vi "Dashboard Main.vi"() -> ()   [LabVIEW 2017]
uses:
  <vilib>/Utility/miscctls.llb/LVRowAndColumnTypeDef.ctl
  <vilib>/event_ctls.llb/eventvkey.ctl
  <vilib>/Rock Robotics/WPI/Dashboard/WPI_DashboardLogging Global.vi
  <vilib>/Utility/inputDevices.llb/joystickAcquire.vi
  <vilib>/Rock Robotics/Network Tables/NT Read Numeric Array.vi
panel:
  in  "Camera Settings Right":T1={"Frame Rate"=30, "Compression"=30, "Size"=1, "DB Camera Config"=FALSE} {"Frame Rate" scale=1.0..30.0; "Compression" scale=100.0..-1.0; "Size" items=["640x480", "320x240", "160x120"]}
  in  "Camera Name Right":string(combo)="No Camera Selection"
  out "Camera Info":cluster{"Mbps LED":bool, "Mbps":dbl, "fps":dbl} {"fps" format="%#.1g"; "Mbps" format="%#.1g"}
  in  "Camera Settings":T1={"Frame Rate"=30, "Compression"=30, "Size"=1, "DB Camera Config"=FALSE} {"Frame Rate" scale=1.0..30.0; "Compression" scale=100.0..-1.0; "Size" items=["640x480", "320x240", "160x120"]}
  in  "TCP":refnum<k5>
  in  "Rec Mode":enum32{"Stop", "Record", "Playback"}(radio)
  out "Robot IP":string
  out "Image Message":string="Timeout in Camera Communications"
  in  "Dashboard Tab":T2(tab)
  in  "Select Auto":string(combo)="Select Autonomous ..."
  out "NT Connection":bool
  out "MotorChart R":cluster{"Numeric":dbl, "Numeric":dbl}(graph)
  out "MotorChart L":cluster{"Numeric":dbl, "Numeric":dbl}(graph)
  out "MotorSliders R":cluster{"MotorSlide1":dbl, "MotorSlide2":dbl} {"MotorSlide2" scale=-1.0..1.0 scale format="%#_2e"; "MotorSlide1" scale=-1.0..1.0 scale format="%#_2e"}
  out "MotorSliders L":cluster{"MotorSlide1":dbl, "MotorSlide2":dbl} {"MotorSlide2" scale=-1.0..1.0 scale format="%#_2e"; "MotorSlide1" scale=-1.0..1.0 scale format="%#_2e"}
  out "Gyro":dbl(knob) scale=0.0..360.0
  out "JS1 Z":dbl(slide) scale=-1.0..1.0 scale format="%#_2e"
  out "JS1 Graph":cluster{"X":dbl, "Y":dbl}[](graph)
  out "JS1 Buttons":T3
  out "JS2 Z":dbl(slide) scale=-1.0..1.0 scale format="%#_2e"
  out "JS2 Graph":cluster{"X":dbl, "Y":dbl}[](graph)
  out "JS2 Buttons":T3
  out "Mode":T4(ring)=enum."Auto Disabled"
  out "Camera Image Right":T5(plugin-control)
  in  "DB/String 9":string
  in  "DB/String 8":string
  in  "DB/String 7":string
  in  "DB/String 6":string
  in  "DB/String 5":string
  in  "DB/String 4":string
  in  "DB/String 3":string
  in  "DB/String 2":string
  in  "DB/String 1":string
  in  "DB/String 0":string
  in  "DB/Slider 0":dbl(slide) scale=0.0..5.0
  in  "DB/Slider 1":dbl(slide) scale=0.0..5.0
  in  "DB/Slider 2":dbl(slide) scale=0.0..5.0
  in  "DB/Slider 3":dbl(slide) scale=0.0..5.0
  out "DB/LED 3":bool
  out "DB/LED 2":bool
  out "DB/LED 1":bool
  out "DB/LED 0":bool
  in  "DB/Button 3":bool
  in  "DB/Button 2":bool
  in  "DB/Button 1":bool
  in  "DB/Button 0":bool caption="New Name"
  in  "Test Slider":dbl(slide) scale=0.0..100.0 scale format="%#_3g"
  in  "On/Off":bool caption="Solenoid"
  in  "Test Name":u16(ring) items=["Select the test to run..."]
  in  "Test Tree":string(tree)
  in  "Motor":cluster{"Value":dbl, "Enable":bool} {"Value" scale=-1.0..1.0 scale format="%#_3g"}
  out "Progress":T6 {"Test Progress" scale=0.0..100.0}
  in  "Rev/Fwd":cluster{"Forward":bool, "Reverse":bool}
  in  "Test Ring":u16(ring) items=["Monochrome", "Color"]
  out "Cmd Status":string
  in  "Execute Command":bool
  in  "Command Params":string[][](table)
  in  "Command Selection":i32(listbox)
  in  "CheckList":i32(listbox)
  out "Tree":string(tree)
  out "Camera Image":T5(plugin-control)
  out "Background":bool
  in  "Camera Name":string(combo)="No Camera Selection"
  # "HW"
  # "HW"
  # "Joysticks"
  # "Drive Motors"
  # "Front"
  # "Right"
  # "Left"
  # "Back"
  # "This tab is a great place for autonomous settings and robot-specific values.\nPlace controls and indicators inside this tab and match name to\nDashboard Variables on robot. You can also delete this comment."
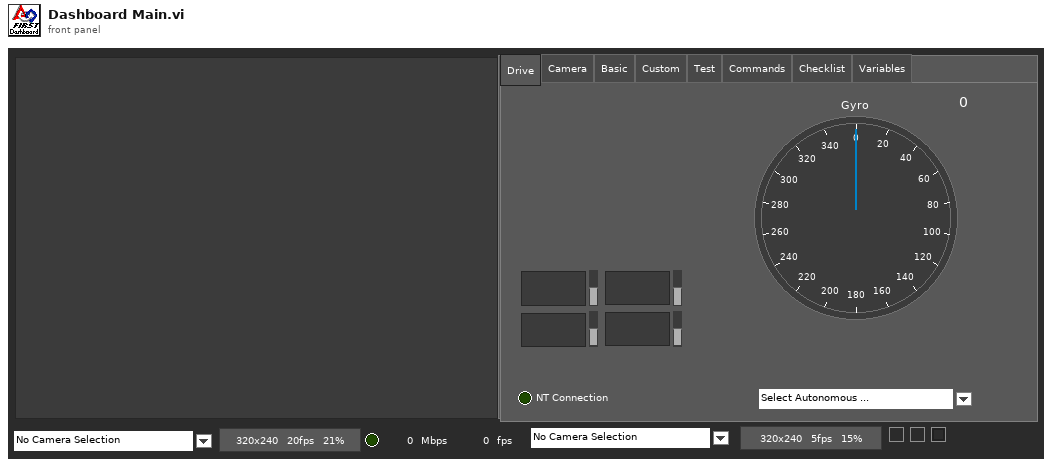
[diagram p1: front panel]
types:
  T1 = cluster{"Frame Rate":i32, "Compression":i32, "Size":u16, "DB Camera Config":bool}
  T2 = enum32{"Drive", "Camera", "Basic", "Custom", "Test", "Commands", "Checklist", "Variables"}
  T3 = cluster{bool, bool, bool, bool, bool, bool, bool, bool, bool, bool, bool, bool}
  T4 = enum8{"Tele-Op Disabled", "Tele-Op Enabled", "Auto Disabled", "Auto Enabled", "Test Disabled", "Test Enabled", "Disconnected", "No Code", "E-Stop"}
  T5 = typedef "IMAQ Image.ctl" = refnum<image>
  T6 = cluster{"Test Progress":u8, "Test Progress Text":string}
  T7 = cluster{"Save Path":path, "Interval (s)":dbl, "Keep":i32}
  T8 = typedef "Image Type" = u32
  T9 = cluster{"IDs":cluster{"RPC field ID":u16, "Unique ID":u16}, "String":string}
  T10 = cluster{"button 1":bool, "button 2":bool, "button 3":bool, "button 4":bool, "button 5":bool, "button 6":bool, "button 7":bool, "button 8":bool, "button 9":bool, "button 10":bool, "button 11":bool, "button 12":bool, "button 13":bool, "button 14":bool, "button 15":bool, "button 16":bool, "button 17":bool, "button 18":bool, "button 19":bool, "button 20":bool, "button 21":bool, "button 22":bool, "button 23":bool, "button 24":bool, "button 25":bool, "button 26":bool, "button 27":bool, "button 28":bool, "button 29":bool, "button 30":bool, "button 31":bool, "button 32":bool}
  T11 = cluster{"Error Strings":string, "Disable Counts":cluster{u16, u16}, "Rail Faults":cluster{u16, u16, u16}, "Robot IP":string, "DB Mode":u8, "Event Info":cluster{"Name":string, "Type":u8, "Number":u16, "Replay":u8}}
  T12 = cluster{"Storage":cluster{"Disk Free":u64, "RAM Block":u32, "RAM free":u32}, "CPU Utilization":cluster{"CPU % ISR":sgl, "CPU % Time Crit":sgl, "CPU % Timed Str":sgl, "CPU % High":sgl, "CPU % Above":sgl, "CPU % Normal":sgl, "CPU % Low":sgl}, "CAN":cluster{"% Bus Utilization":sgl, "Bus Off Cnt":u32, "TX_FIFO Full Cnt":u32, "Receive Error Cnt":u8, "Transmit Error Cnt":u8}, "HID":cluster{"HID Outputs":u32, "Rumble Low":u16, "Rumble High":u16}[]}
  T13 = cluster{"Status bits":cluster{"Test Mode":bool, "Autonomous":bool, "Enabled":bool, "Code Start":bool, "Brownout":bool, "Reserved 2":bool, "Reserved 3":bool, "E-Stop":bool}, "Code Trace":cluster{"Disabled":bool, "TeleOp":bool, "Auto":bool, "Test":bool}, "Controller Type":enum16{"unknown", "cRIO", "roboRio"}, "Code?":enum16{"unknown", "noCode", "code"}, "Battery V":dbl}
  T14 = cluster{"Control Bits":cluster{"TestMode":bool, "Autonomous":bool, "Enabled":bool, "FMS Present":bool, bool, bool, bool, "E-Stop":bool}, "Team Station ":u8, "Countdown":sgl, "Joystick Values":cluster{"Axes":dbl[], "Buttons":bool[], "POVs":i16[]}[]}
  T15 = cluster{"Axes":dbl[], "Buttons":bool[], "POVs":i16[]}[]
  T16 = cluster{"Axes":dbl[], "Buttons":bool[], "POVs":i16[]}
  T17 = cluster{"Buttons[0]":bool, "Buttons[1]":bool, "Buttons[2]":bool, "Buttons[3]":bool, "Buttons[4]":bool, "Buttons[5]":bool, "Buttons[6]":bool, "Buttons[7]":bool, "Buttons[8]":bool, "Buttons[9]":bool, "Buttons[10]":bool, "Buttons[11]":bool}
  T18 = cluster{"Camera Image":refnum<vi>, "Dashboard Tab":refnum<vi>, "Background":refnum<vi>, "Rec Mode":refnum<vi>, "Test Slider":refnum<vi>, "On/Off ":refnum<vi>, "Test Ring":refnum<vi>, "Rev/Fwd":refnum<vi>, "Test Name":refnum<vi>, "Motor":refnum<vi>, "Progress":refnum<vi>, "CheckList":refnum<vi>, "Tree":refnum<vi>, "Test Tree":refnum<vi>, "Command Params":refnum<vi>, "Command Selection":refnum<vi>, "Execute Command":refnum<vi>, "Cmd Status":refnum<vi>, "Camera Settings":refnum<vi>, "Camera Name":refnum<vi>, "Camera Info":refnum<vi>, "Camera Settings Right":refnum<vi>, "Camera Name Right":refnum<vi>, "Camera Image Right":refnum<vi>}
  T19 = cluster{"Camera Name Right":string, string, "Saved DB Images Info":cluster{"Save Path":path, "Interval (s)":dbl, "Keep":i32}}
  T20 = cluster{"Camera Name":string, string, "Saved DB Images Info":cluster{"Save Path":path, "Interval (s)":dbl, "Keep":i32}}
  T21 = cluster{"Operation":enum16{"Update", "Clear"}, "Color Box":u32}[]
  T22 = typedef "eventvkey.ctl" = enum16{"ASCII", "Enter", "Return", "Shift", "Ctrl", "Alt", "Cmd", "Opt", "Caps", "NumLock", "Clear", "Break", "Up", "Down", "Left", "Right", "Insert", "Delete", "Home", "End", "PageUp", "PageDown", "Escape", "Help", "Pause", "ScrollLock", "F1", "F2", "F3", "F4", "F5", "F6", "F7", "F8", "F9", "F10", "F11", "F12", "F13", "F14", "F15", "F16", "F17", "F18", "F19", "F20", "F21", "F22", "F23", "F24", "Play", "VolumeUp", "VolumeDown", "Mute", "Two Byte Char"}
  T23 = cluster{"Image Size":bool, "Image Type":bool, "Pixel Value":bool, "ROI Information":bool, "Zoom Factor":bool}
  T24 = cluster{"Operation":enum16{"Update", "Clear"}, "Color Box":u32}
  T25 = typedef "LVRowAndColumnTypeDef.ctl" = cluster{"Row":i32, "Column":i32}
  T26 = cluster{"Shift":bool, "Ctrl":bool, "Alt":bool, "Cmd":bool, "Opt":bool}
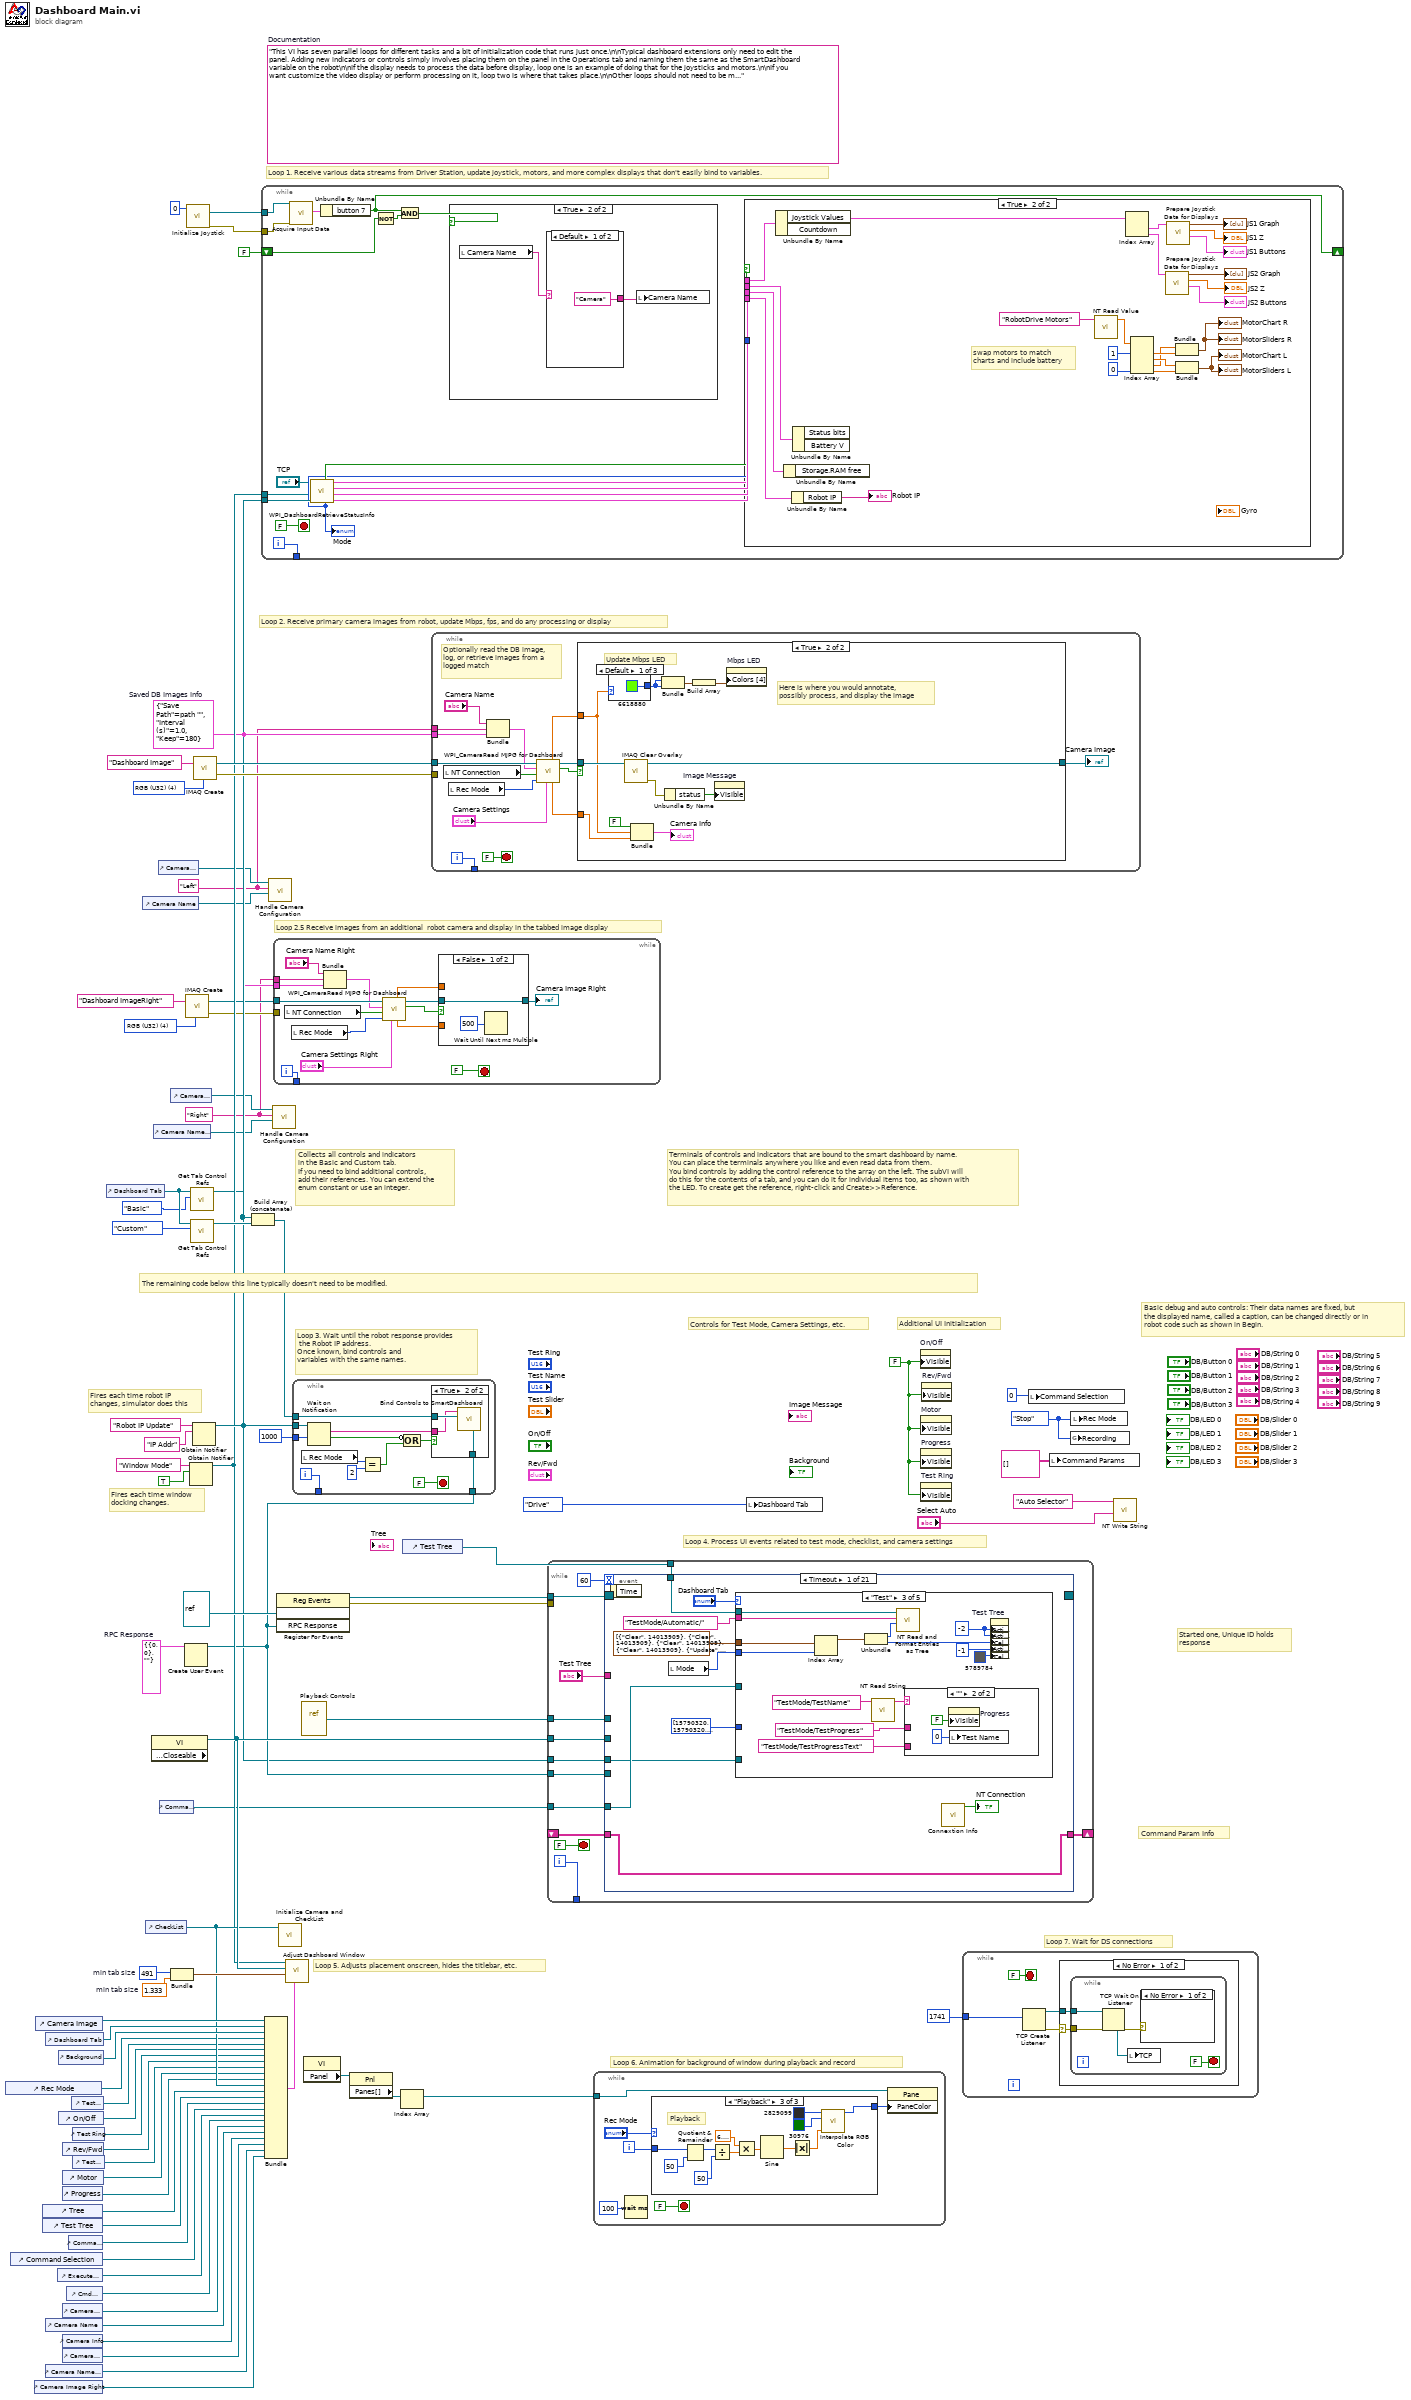
[diagram p0: block diagram]
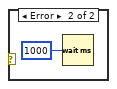
[diagram p3: hidden frame]
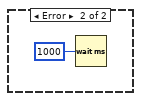
[diagram p4: hidden frame]
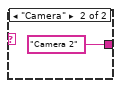
[diagram p6: hidden frame]
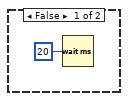
[diagram p7: hidden frame]
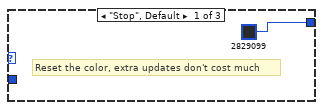
[diagram p8: hidden frame]
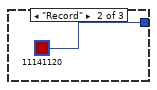
[diagram p9: hidden frame]
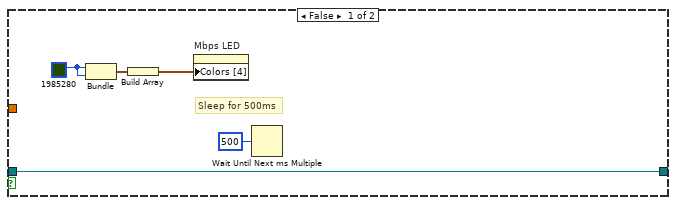
[diagram p11: hidden frame]
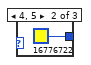
[diagram p12: hidden frame]
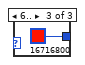
[diagram p13: hidden frame]
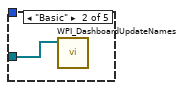
[diagram p15: hidden frame]
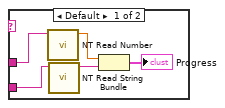
[diagram p16: hidden frame]
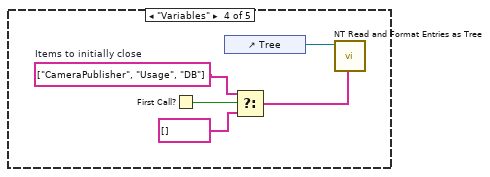
[diagram p17: hidden frame]
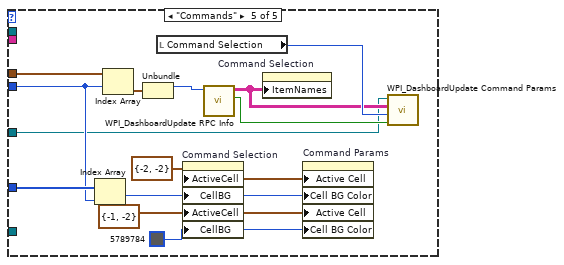
[diagram p18: hidden frame]
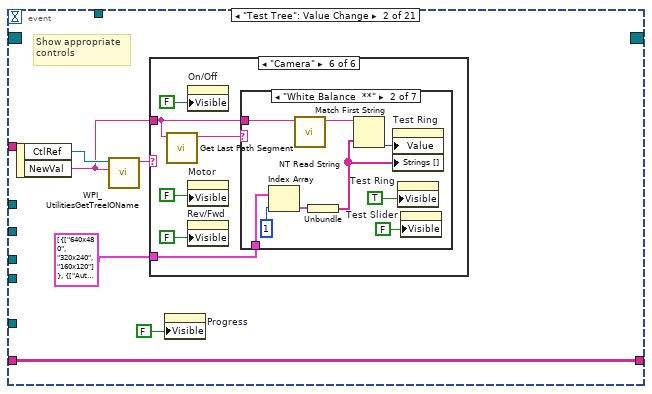
[diagram p19: hidden frame]
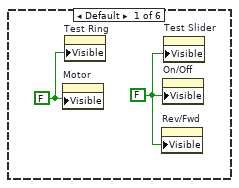
[diagram p20: hidden frame]
diagram:
  w7 = T7 {"Save Path"=path "", "Interval (s)"=1.0, "Keep"=180}  # Saved DB Images Info
  w6 = "Right"
  w5 = "Left"
  w17 = T8 4 items=["Grayscale (U8)", "Grayscale (I16)", "Grayscale (SGL)", "Complex (CSG)", "RGB (U32)", "HSL (U32)", "RGB (U64)"] ("Image Type")
  w33 = T9 {"IDs"={"RPC field ID"=0, "Unique ID"=0}, "String"=""}  # RPC Response
  w56 = 491  # min tab size
  w55 = 1.333  # min tab size
  w63 = enum32{"Stop", "Record", "Playback"}."Stop" ("Rec Mode")
  w40 = FALSE ("Visible")
  (unwired) "This VI has seven parallel loops for different tasks and a bit of initialization code that runs just once.\n\nTypical dashboard extensions only need to edit the panel. Adding new indicators or controls simply involves placing them on the panel in the Operations tab and naming them the same as the SmartDashboard variable on the robot\n\nIf the display needs to process the data before display, loop one is an example of doing that for the joysticks and motors.\n\nIf you want customize the video display or perform processing on it, loop two is where that takes place.\n\nOther loops should not need to be modified. They are pretty standard, and document the task they perform."  # Documentation
  w80 = T8 4 items=["Grayscale (U8)", "Grayscale (I16)", "Grayscale (SGL)", "Complex (CSG)", "RGB (U32)", "HSL (U32)", "RGB (U64)"] ("Image Type")
  # "Loop 2.5 Receive images from an additional  robot camera and display in the tabbed image display"
  # "Command Param Info"
  # "Started one, Unique ID holds\nresponse"
  # "Loop 7. Wait for DS connections"
  # "Basic debug and auto controls: Their data names are fixed, but\nthe displayed name, called a caption, can be changed directly or in\nrobot code such as shown in Begin."
  # "Controls for Test Mode, Camera Settings, etc."
  # "Additional UI Initialization"
  # "Loop 6. Animation for background of window during playback and record"
  # "Fires each time robot IP\nchanges, simulator does this"
  # "Fires each time window\ndocking changes."
  # "Collects all controls and indicators\nin the Basic and Custom tab.\nIf you need to bind additional controls,\nadd their references. You can extend the\nenum constant or use an integer."
  # "The remaining code below this line typically doesn't need to be modified."
  # "Loop 4. Process UI events related to test mode, checklist, and camera settings"
  # "Terminals of controls and indicators that are bound to the smart dashboard by name.\nYou can place the terminals anywhere you like and even read data from them.\nYou bind controls by adding the control reference to the array on the left. The subVI will\ndo this for the contents of a tab, and you can do it for individual items too, as shown with\nthe LED. To create get the reference, right-click and Create>>Reference."
  # "Loop 3. Wait until the robot response provides\n the Robot IP address.\nOnce known, bind controls and\nvariables with the same names."
  # "Loop 5. Adjusts placement onscreen, hides the titlebar, etc."
  # "Loop 1. Receive various data streams from Driver Station, update joystick, motors, and more complex displays that don't easily bind to variables."
  # "Loop 2. Receive primary camera images from robot, update Mbps, fps, and do any processing or display"
  n1 = control-ref of="Rec Mode"() -> (w46:refnum<vi>)
  n2 = control-ref of="Command Selection"() -> (w32:refnum<vi>)
  n3 = control-ref of="Camera Image Right"() -> (w10:refnum<vi>)
  n4 = control-ref of="Camera Image"() -> (w58:refnum<vi>)
  n5 = control-ref of="Tree"() -> (w50:refnum<vi>)
  n6 = control-ref of="Test Tree"() -> (w49:refnum<vi>)
  n7 = control-ref of="Dashboard Tab"() -> (w57:refnum<vi>)
  n8 = control-ref of="Camera Name"() -> (w23:refnum<vi>)
  n9 = control-ref of="Camera Name Right"() -> (w11:refnum<vi>)
  n10 = control-ref of="Execute Command"() -> (w34:refnum<vi>)
  n11 = control-ref of="Background"() -> (w53:refnum<vi>)
  n12 = control-ref of="On/Off"() -> (w44:refnum<vi>)
  n13 = control-ref of="Progress"() -> (w41:refnum<vi>)
  n14 = control-ref of="Camera Settings"() -> (w24:refnum<vi>)
  n15 = control-ref of="Camera Info"() -> (w22:refnum<vi>)
  n16 = control-ref of="Camera Settings Right"() -> (w12:refnum<vi>)
  n17 = control-ref of="Rev/Fwd"() -> (w42:refnum<vi>)
  n18 = control-ref of="Motor"() -> (w47:refnum<vi>)
  n19 = control-ref of="Cmd Status"() -> (w28:refnum<vi>)
  n20 = control-ref of="Command Params"() -> (w35:refnum<vi>)
  n21 = control-ref of="Test Slider"() -> (w45:refnum<vi>)
  n22 = control-ref of="Test Ring"() -> (w43:refnum<vi>)
  n23 = control-ref of="Test Name"() -> (w48:refnum<vi>)
  n24 = control-ref of="Dashboard Tab"() -> (w61:refnum<vi>)
  n25 = control-ref of="Camera Name"() -> (w25:refnum<vi>)
  n26 = control-ref of="CheckList"() -> (w51:refnum<vi>)
  n27 = property class="VI" props=["Front Panel.Closeable"]() -> (reference out=w62:refnum<vi>)  [unwired: 2 in, 2 out]
  n28 = control-ref of="Camera Name Right"() -> (w13:refnum<vi>)
  n29 = control-ref of="Camera Settings"() -> (w26:refnum<vi>)
  n30 = control-ref of="Command Params"() -> (w27:refnum<vi>)
  n31 = control-ref of="Camera Settings Right"() -> (w14:refnum<vi>)
  n32 = Bundle("min tab size"=w56, "min tab size"=w55) -> (w54:cluster{"min tab size":i32, "min tab size":dbl})  [unwired: 1 in]
  n33 = Create User Event(user event datatype=w33) -> (user event=w29:refnum<user-event>)  [unwired: 1 in, 1 out]
  n34 = call "IMAQ Create"("Image Name"="Dashboard ImageRight", "Image Type"=w17) -> ("New Image"=w16:T5, "error out"=w15:errorcluster)  [unwired: 2 in, 1 out]
  n35 = call <vilib>:"Initialize Joystick.vi"("device index"=0) -> ("error out"=w3:errorcluster, "device ID"=w4:refnum<k1>)  [unwired: 9 in]
  n36 = Obtain Notifier(name (unnamed)="Window Mode", notification data type=TRUE) -> (notifier out=w38:refnum<notifier>)  [unwired: 2 in, 2 out]
  n37 = call <vilib>:"Get Tab Control Refs.vi"("Page Index"=T2."Basic" ("Dashboard Tab"), "TabControl in"=w61) -> ("ControlsOnPage"=w21:refnum<vi>[])  [unwired: 9 in]
  n38 = call <vilib>:"Get Tab Control Refs.vi"("Page Index"=T2."Custom" ("Dashboard Tab"), "TabControl in"=w61) -> ("ControlsOnPage"=w60:refnum<vi>[])  [unwired: 9 in]
  n39 = Obtain Notifier(name (unnamed)="Robot IP Update", notification data type="IP Addr" ("name (unnamed)")) -> (notifier out=w39:refnum<notifier>)  [unwired: 2 in, 2 out]
  n40 = call "IMAQ Create"("Image Name"="Dashboard Image", "Image Type"=w80) -> ("New Image"=w78:T5, "error out"=w77:errorcluster)  [unwired: 2 in, 1 out]
  n41 = Build Array (concatenate)(w21, w60) -> (w59:refnum<vi>[])
  n42 = while {
    tunnel: [w97] -> _
    tunnel: w39 -> [w91]
    tunnel: w38 -> [w88]
    tunnel: w4 -> [w87]
    tunnel: w3 -> [w86]
    shift-right: [w84] -> _
    shift-left: FALSE -> [w83]
    i -> [w97]
    stop <- FALSE stop-if-true
    n43 = call-poly <vilib>:"Acquire Input Data.vi"("device ID"=w87, "error in (no error)"=w86) -> ("button info"=w85:T10)  [unwired: 13 in, 4 out]
    n44 = call <vilib>:"WPI_DashboardRetrieveStatusInfo.vi"("Binding Refnum"=w91, "Window Mode Notifier"=w88, "TCP Cnx"="TCP") -> ("Power and Errors"=w92:T11, "Robot Metrics"=w95:T12, "Status Info"=w96:T13, "Control Info"=w93:T14, "Robot Mode"=w90:T4, "Process?"=w94:bool)  [unwired: 3 in]
    "Mode" <- w90
    n45 = Unbundle By Name(w85) -> ("button 7"=w84:bool)
    n46 = Not(x=w83) -> (.not. x?=w82:bool)
    n47 = And(x=w84, y=w82) -> (x .and. y?=w81:bool)
    n48 = case shown="True" w81 {
      frame False {
      }
      frame True {
        n49 = local read "Camera Name"() -> (w100:string)
        n50 = case shown="Default" w100 {
          tunnel: ["Camera" "Camera 2"] -> w99
          frame Default {
          }
          frame "Camera" {
          }
        }
        n51 = local write "Camera Name"(w99) -> ()
      }
    }
    n52 = case shown="True" w94 {
      tunnel: w96 -> [_ w127]
      tunnel: w95 -> [_ w126]
      tunnel: w93 -> [_ w125]
      tunnel: w92 -> [_ w124]
      tunnel: w90 -> [_ _]
      frame False {
        n53 = Wait (ms)(milliseconds to wait=u32 20) -> ()  [unwired: 1 out]
      }
      frame True {
        # "swap motors to match\ncharts and include battery"
        n54 = Unbundle By Name(w125) -> ("Joystick Values"=w115:T15)  [unwired: 1 out]
        n55 = Unbundle By Name(w126) -> ()  [unwired: 1 out]
        n56 = Unbundle By Name(w124) -> ("Robot IP"=→"Robot IP":string)
        n57 = Unbundle By Name(w127) -> ()  [unwired: 2 out]
        n58 = call-poly <vilib>:"NT Read Value.vi"("Name"="RobotDrive Motors") -> ("Numeric Array"=w105:dbl[])  [unwired: 9 in, 1 out]
        n59 = Index Array(array=w115) -> (element #1=w114:T16, element #2=w110:T16)  [unwired: 2 in]
        n60 = Index Array(array=w105, index #1=1, index #4=0) -> (element #1=w119:dbl, element #2=w120:dbl, element #3=w118:dbl, element #4=w123:dbl)  [unwired: 2 in]
        n61 = call "Prepare Joystick Data for Displays.vi"("Joystick Values"=w110) -> ("Buttons"=→"JS2 Buttons":T17, "Z Axis"=→"JS2 Z":dbl, "Cartesian Data"=→"JS2 Graph":cluster{"X axis":dbl, "X axis":dbl}[])  [unwired: 8 in]
        n62 = call "Prepare Joystick Data for Displays.vi"("Joystick Values"=w114) -> ("Buttons"=→"JS1 Buttons":T17, "Z Axis"=→"JS1 Z":dbl, "Cartesian Data"=→"JS1 Graph":cluster{"X axis":dbl, "X axis":dbl}[])  [unwired: 8 in]
        n63 = Bundle("Numeric"=w118, "Numeric"=w119) -> (→"MotorChart R" →"MotorSliders R":cluster{"Numeric":dbl, "Numeric":dbl})  [unwired: 1 in]
        n64 = Bundle("Numeric"=w120, "Numeric"=w123) -> (→"MotorChart L" →"MotorSliders L":cluster{"Numeric":dbl, "Numeric":dbl})  [unwired: 1 in]
      }
    }
  }
  n65 = Bundle("Camera Image"=w58, "Dashboard Tab"=w57, "Background"=w53, "Rec Mode"=w46, "Test Slider"=w45, "On/Off"=w44, "Test Ring"=w43, "Rev/Fwd"=w42, "Test Name"=w48, "Motor"=w47, "Progress"=w41, "CheckList"=w51, "Tree"=w50, "Test Tree"=w49, "Command Params"=w35, "Command Selection"=w32, "Execute Command"=w34, "Cmd Status"=w28, "Camera Settings"=w24, "Camera Name"=w23, "Camera Info"=w22, "Camera Settings Right"=w12, "Camera Name Right"=w11, "Camera Image Right"=w10) -> (w52:T18)  [unwired: 1 in]
  n66 = call "Handle Camera Configuration.vi"("CameraNameRef"=w25, "Display Name"=w5, "ClusterRef"=w26) -> ()  [unwired: 9 in]
  n67 = call "Handle Camera Configuration.vi"("CameraNameRef"=w13, "Display Name"=w6, "ClusterRef"=w14) -> ()  [unwired: 9 in]
  n68 = while {
    tunnel: w16 -> [w142]
    tunnel: w15 -> [_]
    tunnel: [w137] -> _
    tunnel: w7 -> [w131]
    tunnel: w6 -> [w128]
    i -> [w137]
    stop <- FALSE stop-if-true
    n69 = local read "NT Connection"() -> (w132:bool)
    n70 = local read "Rec Mode"() -> (w141:enum32{"Stop", "Record", "Playback"})
    n71 = Bundle("Camera Name Right"="Camera Name Right", w128, "Saved DB Images Info"=w131) -> (w130:T19)  [unwired: 1 in]
    n72 = call <vilib>:"WPI_CameraRead MJPG for Dashboard.vi"("Camera Settings"="Camera Settings Right", "Rec Mode"=w141, "NT Connection"=w132, "Capture Info"=w130, "Refnum in"=w142) -> ("Active"=w136:bool, "Refnum out"=w139:T5, "FPS"=w134:dbl, "Bandwidth (Mbps)"=w135:dbl)  [unwired: 3 in]
    n73 = case shown="False" w136 {
      tunnel: w139 -> [w143 w145]
      tunnel: w135 -> [_ _]
      tunnel: w134 -> [_ _]
      tunnel: [w143 w145] -> w133
      frame False {
        n74 = Wait Until Next ms Multiple(millisecond multiple=u32 500) -> ()  [unwired: 1 out]
      }
      frame True {
      }
    }
    "Camera Image Right" <- w133
  }
  n75 = register-events(refnum<vi> refnum, w29) -> (reference out=w67:refnum<event-registration>, error out=w66:errorcluster)  [unwired: 2 in]
  n76 = call "Initialize Camera and CheckList.vi"("ListBox in"=w51) -> ()  [unwired: 11 in]
  n77 = call "Adjust Dashboard Window.vi"("Sizing Refnums"=w52, "Size Constraints"=w54, "VI"=w62, "WIn Mode"=w38) -> ()  [unwired: 8 in]
  n78 = while {
    tunnel: w59 -> [w157]
    tunnel: w39 -> [w155]
    tunnel: [w153] -> _
    tunnel: u32 1000 ("milliseconds to wait") -> [w152]
    tunnel: w29 -> [w146]
    i -> [w153]
    stop <- FALSE stop-if-true
    n79 = local read "Rec Mode"() -> (w148:enum32{"Stop", "Record", "Playback"})
    n80 = Wait on Notification(notifier=w155, timeout in ms (-1)=w152) -> (notification=w154:string, timed out?=w150:bool)  [unwired: 2 in, 2 out]
    n81 = Equal?(x=w148, y=u16 2 ("Rec Mode")) -> (x = y?=w149:bool)
    n82 = Compound Arithmetic op=OR(invert w150, w149) -> (w151:bool)
    n83 = case shown="True" w151 {
      tunnel: w157 -> [_ w160]
      tunnel: w154 -> [_ w159]
      tunnel: w146 -> [_ w158]
      frame False {
      }
      frame True {
        n84 = call <vilib>:"Bind Controls to SmartDashboard.vi"("RPC ref"=w158, "Bound Control Refs"=w160, "Server IP Address"=w159) -> ()  [unwired: 9 in]
      }
    }
  }
  n85 = vi-ref "Playback Controls.vi"() -> (w68:refnum<vi>)
  n86 = property class="VI"() -> ("Panel"=w70:refnum<vi>)  [unwired: 2 in, 2 out]
  n87 = property class="Pnl"(reference=w70) -> ("Panes[]"=w71:refnum<vi>[])  [unwired: 1 in, 2 out]
  n88 = Index Array(array=w71) -> (element=w69:refnum<vi>)  [unwired: 1 in]
  n89 = control-ref of="Test Tree"() -> (w72:refnum<vi>)
  n90 = while {
    tunnel: w78 -> [w173]
    tunnel: w77 -> [_]
    tunnel: [w174] -> _
    tunnel: w7 -> [w164]
    tunnel: w5 -> [w161]
    i -> [w174]
    stop <- FALSE stop-if-true
    # "Optionally read the DB image,\nlog, or retrieve images from a\nlogged match"
    n91 = local read "NT Connection"() -> (w165:bool)
    n92 = local read "Rec Mode"() -> (w169:enum32{"Stop", "Record", "Playback"})
    n93 = Bundle("Camera Name"="Camera Name", w161, "Saved DB Images Info"=w164) -> (w163:T20)  [unwired: 1 in]
    n94 = call <vilib>:"WPI_CameraRead MJPG for Dashboard.vi"("Camera Settings"="Camera Settings", "Rec Mode"=w169, "NT Connection"=w165, "Capture Info"=w163, "Refnum in"=w173) -> ("Active"=w171:bool, "Refnum out"=w172:T5, "FPS"=w170:dbl, "Bandwidth (Mbps)"=w168:dbl)  [unwired: 3 in]
    n95 = case shown="True" w171 {
      tunnel: w172 -> [w176 w187]
      tunnel: w168 -> [_ w184]
      tunnel: w170 -> [_ w185]
      tunnel: [w176 w181] -> w166
      frame False {
        w178 = u32 1985280 ("Color Box")
        # "Sleep for 500ms"
        n96 = Bundle("Color Box"=w178, "Color Box"=w178) -> (w179:cluster{"Color Box":u32, "Color Box":u32})  [unwired: 1 out]
        n97 = Build Array(w179) -> (w177:cluster{"Color Box":u32, "Color Box":u32}[])
        n98 = property on="Mbps LED" class="Bool (strict)"("Colors [4]"=w177) -> ()  [unwired: 2 in, 2 out]
        n99 = Wait Until Next ms Multiple(millisecond multiple=u32 500) -> ()  [unwired: 1 out]
      }
      frame True {
        # "Here is where you would annotate,\npossibly process, and display the image"
        # "Update Mbps LED"
        n100 = case shown="Default" w184 {
          tunnel: [u32 6618880 ("Color Box") u32 16776722 ("Color Box") u32 16716800 ("Color Box")] -> w188
          frame Default {
          }
          frame 4, 5 {
          }
          frame 6.. {
          }
        }
        n101 = call "IMAQ Clear Overlay"("Image"=w187) -> ("error out"=w190:errorcluster, "Image Out"=w181:T5)  [unwired: 2 in, 7 out]
        n102 = Bundle(FALSE, "Bandwidth (Mbps)"=w184, "FPS"=w185) -> (→"Camera Info":cluster{bool, "Bandwidth (Mbps)":dbl, "FPS":dbl})  [unwired: 1 in]
        n103 = Bundle("Color Box"=w188, "Color Box"=w188) -> (w189:cluster{"Color Box":u32, "Color Box":u32})  [unwired: 1 out]
        n104 = Unbundle By Name(w190) -> ("status"=w191:bool)
        n105 = Build Array(w189) -> (w186:cluster{"Color Box":u32, "Color Box":u32}[])
        n106 = property on="Image Message" class="Str"("Visible"=w191) -> ()  [unwired: 2 in, 2 out]
        n107 = property on="Mbps LED" class="Bool (strict)"("Colors [4]"=w186) -> ()  [unwired: 2 in, 2 out]
      }
    }
    "Camera Image" <- w166
  }
  n108 = while {
    tunnel: [w204] -> _
    tunnel: w72 -> [w203]
    tunnel: w68 -> [w202]
    tunnel: w67 -> [w201]
    tunnel: w66 -> [_]
    tunnel: w62 -> [w200]
    tunnel: w29 -> [w199]
    tunnel: w27 -> [w198]
    shift-right: [w197] -> _
    shift-left: _ -> [w196]
    tunnel: w21 -> [w195]
    i -> [w204]
    stop <- FALSE stop-if-true
    n109 = event shown="[0] Timeout" {
      selector: w201 -> [_ _ _ _ _ _ _ _ _ _ _ _ _ _ _ _ _ _ _ _ _]
      dyn-events: [_ _ _ _ _ _ _ _ _ _ _ _ _ _ _ _ w464 _ _ _ _] -> _
      timeout: u32 60 ("milliseconds to wait") -> [_ _ _ _ _ _ _ _ _ _ _ _ _ _ _ _ _ _ _ _ _]
      tunnel: w203 -> [w216 _ _ _ _ _ _ _ _ _ _ _ _ _ _ _ _ _ _ _ _]
      tunnel: "Test Tree" -> [_ _ _ _ _ _ _ _ _ _ _ w431 w439 w441 w445 w453 _ _ _ _ _]
      tunnel: w202 -> [_ _ _ _ _ _ _ _ _ _ _ _ _ _ _ _ w466 _ w484 _ _]
      tunnel: w200 -> [_ _ _ _ _ _ _ _ _ _ _ _ _ _ _ _ w462 _ _ _ _]
      tunnel: w199 -> [_ _ _ _ _ _ _ _ _ _ _ _ _ _ _ _ w460 _ _ _ _]
      tunnel: w198 -> [w211 _ _ _ _ _ w382 _ _ _ _ _ _ _ _ _ _ _ _ _ _]
      tunnel: [w210 w259 w361 w366 w375 w379 w380 w389 w399 w406 w418 w430 w437 w440 w444 w452 w459 w479 w481 w485 w498] -> w197
      tunnel: w196 -> [w210 w259 w361 w366 w375 w379 w380 _ _ w406 w418 w430 w437 w440 w444 w452 w459 w479 w481 w485 w498]
      tunnel: w195 -> [w208 _ _ _ _ _ _ _ _ _ _ _ _ _ _ _ _ _ _ _ _]
      event Timeout {
        n110 = event-data() -> ()  [unwired: 1 in, 1 out]
        n111 = local read "Mode"() -> (w213:T4)
        n112 = case shown="\"Test\"" "Dashboard Tab" {
          tunnel: w216 -> [_ _ w232 _ _]
          tunnel: "TestMode/Automatic/" ("Name Pattern") -> [_ _ w231 _ _]
          tunnel: T21 [{"Operation"=enum."Clear", "Color Box"=14013909}, {"Operation"=enum."Clear", "Color Box"=14013909}, {"Operation"=enum."Clear", "Color Box"=14013909}, {"Operation"=enum."Clear", "Color Box"=14013909}, {"Operation"=enum."Update", "Color Box"=14013909}, {"Operation"=enum."Update", "Color Box"=16777215}, {"Operation"=enum."Clear", "Color Box"=14013909}, {"Operation"=enum."Clear", "Color Box"=14013909}, {"Operation"=enum."Clear", "Color Box"=14013909}] -> [_ _ w224 _ w252]
          tunnel: w213 -> [_ _ w223 _ w251]
          tunnel: u32[] [15790320, 15790320, 15790320, 15790320, 16777215, 16777215, 15790320, 15790320, 15790320] -> [_ _ _ _ w257]
          tunnel: w211 -> [_ _ _ _ w245]
          tunnel: w208 -> [_ w218 _ _ _]
          frame "Custom", Default {
          }
          frame "Basic" {
            n113 = call <vilib>:"WPI_DashboardUpdateNames.vi"("Controls on Tab"=w218) -> ()  [unwired: 11 in]
          }
          frame "Test" {
            w230 = -2 ("Active Item:Row Number")
            n114 = Index Array(array=w224, index=w223) -> (element=w225:T24)
            n115 = Unbundle(w225) -> ("Operation"=w226:enum16{"Update", "Clear"}, "Color Box"=w227:u32)
            n116 = call <vilib>:"NT Read String.vi"("Name"="TestMode/TestName") -> ("String"=w221:string)  [unwired: 9 in, 1 out]
            n117 = call <vilib>:"NT Read and Format Entries as Tree.vi"("Operation"=w226, "Name Pattern"=w231, "Tree Refnum"=w232) -> ()  [unwired: 7 in, 2 out]
            n118 = case shown="\"\"" w221 {
              tunnel: "TestMode/TestProgress" ("Name") -> [w234 _]
              tunnel: "TestMode/TestProgressText" ("Name") -> [w233 _]
              frame Default {
                n119 = call <vilib>:"NT Read Number.vi"("Name"=w234) -> ("Numeric"=w235:dbl)  [unwired: 9 in, 1 out]
                n120 = call <vilib>:"NT Read String.vi"("Name"=w233) -> ("String"=w236:string)  [unwired: 9 in, 1 out]
                n121 = Bundle("Numeric"=w235, "String"=w236) -> (→"Progress":cluster{"Numeric":dbl, "String":string})  [unwired: 1 in]
              }
              frame "" {
                n122 = property on="Progress" class="Clust (strict)"("Visible"=FALSE) -> ()  [unwired: 2 in, 2 out]
                n123 = local write "Test Name"(u16 0) -> ()
              }
            }
            n124 = property on="Test Tree" class="Tree (strict)"("Active Item Row Number"=w230, "ActiveColNum"=w230, "CellBG"=w227, "Active Item Row Number"=-1 ("Active Item:Row Number"), "CellBG"=u32 5789784 ("Color Box")) -> ()  [unwired: 2 in, 2 out]
          }
          frame "Variables" {
            w242 = string[] ["CameraPublisher", "Usage", "DB"]  # Items to initially close
            n125 = First Call?() -> (First Call?: T/F=w243:bool)
            n126 = control-ref of="Tree"() -> (w244:refnum<vi>)
            n127 = Select(t=w242, s=w243, f=string[] []) -> (s? t:f=w240:string[])
            n128 = call <vilib>:"NT Read and Format Entries as Tree.vi"("Tags to  Close"=w240, "Tree Refnum"=w244) -> ()  [unwired: 8 in, 2 out]
          }
          frame "Commands" {
            w253 = u32 5789784 ("Color Box")
            w254 = T25 {"Row"=-1, "Column"=-2} ("Active Cell:Active Cell")
            w256 = T25 {"Row"=-2, "Column"=-2} ("Active Cell:Active Cell")
            n129 = Index Array(array=w257, index=w251) -> (element=w255:u32)
            n130 = Index Array(array=w252, index=w251) -> (element=w250:T24)
            n131 = Unbundle(w250) -> ("Operation"=w249:enum16{"Update", "Clear"})  [unwired: 1 out]
            n132 = local read "Command Selection"() -> (w248:i32)
            n133 = property on="Command Selection" class="MCListbox (strict)"("ActiveCell"=w256, "CellBG"=w255, "ActiveCell"=w254, "CellBG"=w253) -> ()  [unwired: 2 in, 2 out]
            n134 = call <vilib>:"WPI_DashboardUpdate RPC Info.vi"("Operation"=w249) -> ("update"=w247:bool, "commands"=w246:string[][])  [unwired: 9 in]
            n135 = property on="Command Selection" class="MCListbox (strict)"("ItemNames"=w246) -> ()  [unwired: 2 in, 2 out]
            n136 = property on="Command Params" class="Tbl (strict)"("Active Cell"=w256, "Cell BG Color"=w255, "Active Cell"=w254, "Cell BG Color"=w253) -> ()  [unwired: 2 in, 2 out]
            n137 = call <vilib>:"WPI_DashboardUpdate Command Params.vi"("Update"=w247, "NewVal"=w248, "Commands"=w246, "Param Tbl"=w245) -> ()  [unwired: 7 in, 1 out]
          }
        }
        n138 = call <vilib>:"Connextion Info.vi"() -> ("Connected"=→"NT Connection":bool)  [unwired: 10 in, 1 out]
      }
      event "Test Tree": Value Change {
        # "Show appropriate\ncontrols"
        n139 = event-data() -> ("CtlRef"=w262:refnum<vi>, "NewVal"=w260:string)  [unwired: 1 in]
        n140 = call <vilib>:"WPI_UtilitiesGetTreeIOName.vi"("NewVal"=w260, "TreeControl in"=w262) -> ("I/O Name"=w263:string)  [unwired: 9 in]
        n141 = case shown="\"Camera\"" w263 {
          selector: w263 -> [_ w270 _ w292 w301 _]
          tunnel: w260 -> [_ _ w289 w291 _ w308]
          tunnel: cluster{string[]}[] [{["640x480", "320x240", "160x120"]}, {["Auto", "Fixed indoor", "Fixed outdoor 1", "Fixed outdoor 2", "Fixed fluorescent 1", "Fixed fluorescent 2", "Hold current"]}, {["Auto", "Flicker-free 50 Hz", "Flicker-free 60 Hz", "Hold current"]}, {["None", "Prioritize frame rate", "Prioritize image quality"]}, {["Monochrome", "Color"]}] -> [_ _ _ _ _ w307]
          frame Default {
            w265 = FALSE ("Visible")
            w264 = FALSE ("Visible")
            n142 = property on="Motor" class="Clust (strict)"("Visible"=w264) -> ()  [unwired: 2 in, 2 out]
            n143 = property on="Test Ring" class="Ring (strict)"("Visible"=w264) -> ()  [unwired: 2 in, 2 out]
            n144 = property on="Rev/Fwd" class="Clust (strict)"("Visible"=w265) -> ()  [unwired: 2 in, 2 out]
            n145 = property on="On/Off" class="Bool (strict)"("Visible"=w265) -> ()  [unwired: 2 in, 2 out]
            n146 = property on="Test Slider" class="Slide (strict)"("Visible"=w265) -> ()  [unwired: 2 in, 2 out]
          }
          frame "Analog Out", "Motor", "PWM" {
            w271 = FALSE ("Visible")
            n147 = case shown="\"Analog Out\"" w270 {
              tunnel: [1.0 ("Value") -1.0 ("Value") 0.0 ("Value")] -> w269
              tunnel: [255.0 ("Value") 1.0 ("Value") 5.0 ("Value")] -> w268
              tunnel: [128.0 ("Value") 0.0 ("Value") 0.0 ("Value")] -> w267
              tunnel: [64.0 ("Value") 0.5 ("Value") 1.0 ("Value")] -> w266
              frame "PWM" {
              }
              frame "Motor", Default {
              }
              frame "Analog Out" {
              }
            }
            n148 = property on="Motor" class="Clust (strict)"("Visible"=TRUE) -> ()  [unwired: 2 in, 2 out]
            n149 = property on="Value" class="Slide (strict)"("Value"=w267, "Scale.Minimum"=w269, "Scale.Maximum"=w268, "Scale.Increment"=w266) -> ()  [unwired: 2 in, 2 out]
            n150 = property on="On/Off" class="Bool (strict)"("Visible"=w271) -> ()  [unwired: 2 in, 2 out]
            n151 = property on="Test Slider" class="Slide (strict)"("Visible"=w271) -> ()  [unwired: 2 in, 2 out]
            n152 = property on="Test Ring" class="Ring (strict)"("Visible"=w271) -> ()  [unwired: 2 in, 2 out]
            n153 = property on="Rev/Fwd" class="Clust (strict)"("Visible"=w271) -> ()  [unwired: 2 in, 2 out]
          }
          frame "Servo" {
            w287 = FALSE ("Visible")
            n154 = call <vilib>:"NT Read Number.vi"("Name"=w289) -> ("Numeric"=w288:dbl)  [unwired: 9 in, 1 out]
            n155 = property on="Test Slider" class="Slide (strict)"("Visible"=TRUE, "Scale.Maximum"=170.0 ("Scale.Range:Maximum")) -> ()  [unwired: 2 in, 2 out]
            n156 = local write "Test Slider"(w288) -> ()
            n157 = property on="Motor" class="Clust (strict)"("Visible"=w287) -> ()  [unwired: 2 in, 2 out]
            n158 = property on="Rev/Fwd" class="Clust (strict)"("Visible"=w287) -> ()  [unwired: 2 in, 2 out]
            n159 = property on="On/Off" class="Bool (strict)"("Visible"=w287) -> ()  [unwired: 2 in, 2 out]
            n160 = property on="Test Ring" class="Ring (strict)"("Visible"=w287) -> ()  [unwired: 2 in, 2 out]
          }
          frame "Relay", "Solenoid" {
            w290 = FALSE ("Visible")
            n161 = property on="Motor" class="Clust (strict)"("Visible"=w290) -> ()  [unwired: 2 in, 2 out]
            n162 = property on="Test Slider" class="Slide (strict)"("Visible"=w290) -> ()  [unwired: 2 in, 2 out]
            n163 = Search and Replace String(input string=w291, search string="/Value  **", replace string="/Direction") -> (result string=w297:string)  [unwired: 5 in, 3 out]
            n164 = property on="Test Ring" class="Ring (strict)"("Visible"=w290) -> ()  [unwired: 2 in, 2 out]
            n165 = call <vilib>:"NT Read String.vi"("Name"=w297) -> ("String"=w295:string)  [unwired: 9 in, 1 out]
            n166 = Equal?(x="Both directions", y=w295) -> (x = y?=w293:bool)
            n167 = Not(x=w293) -> (.not. x?=w294:bool)
            n168 = property on="Rev/Fwd" class="Clust (strict)"("Visible"=w293) -> ()  [unwired: 2 in, 2 out]
            n169 = property on="On/Off" class="Bool (strict)"("Visible"=w294, "Caption.Text"=w292) -> ()  [unwired: 2 in, 2 out]
          }
          frame "Compressor", "Digital Out" {
            w300 = FALSE ("Visible")
            # "Get direction and finish"
            n170 = property on="Motor" class="Clust (strict)"("Visible"=w300) -> ()  [unwired: 2 in, 2 out]
            n171 = property on="Test Slider" class="Slide (strict)"("Visible"=w300) -> ()  [unwired: 2 in, 2 out]
            n172 = property on="Test Ring" class="Ring (strict)"("Visible"=w300) -> ()  [unwired: 2 in, 2 out]
            n173 = property on="On/Off" class="Bool (strict)"("Visible"=TRUE, "Caption.Text"=w301) -> ()  [unwired: 2 in, 2 out]
            n174 = property on="Rev/Fwd" class="Clust (strict)"("Visible"=FALSE) -> ()  [unwired: 2 in, 2 out]
          }
          frame "Camera" {
            n175 = call <vilib>:"Get Last Path Segment.vi"("String in"=w308) -> ("String out"=w309:string)  [unwired: 10 in]
            n176 = property on="On/Off" class="Bool (strict)"("Visible"=FALSE) -> ()  [unwired: 2 in, 2 out]
            n177 = property on="Motor" class="Clust (strict)"("Visible"=FALSE) -> ()  [unwired: 2 in, 2 out]
            n178 = property on="Rev/Fwd" class="Clust (strict)"("Visible"=FALSE) -> ()  [unwired: 2 in, 2 out]
            n179 = case shown="\"White Balance  **\"" w309 {
              tunnel: w308 -> [w315 w324 w333 w342 w351 _ w357]
              tunnel: w307 -> [w313 w321 w330 w339 w348 _ _]
              frame "Size  **" {
                n180 = Index Array(array=w313) -> (element=w312:cluster{string[]})  [unwired: 1 in]
                n181 = call <vilib>:"NT Read String.vi"("Name"=w315) -> ("String"=w314:string)  [unwired: 9 in, 1 out]
                n182 = Unbundle(w312) -> (w310:string[])
                n183 = Match First String(2:w310, 3:w314) -> (0:w311:i32)  [unwired: 1 out]
                n184 = property on="Test Ring" class="Ring (strict)"("Value"=w311, "Strings []"=w310) -> ()  [unwired: 2 in, 2 out]
                n185 = property on="Test Ring" class="Ring (strict)"("Visible"=TRUE) -> ()  [unwired: 2 in, 2 out]
                n186 = property on="Test Slider" class="Slide (strict)"("Visible"=FALSE) -> ()  [unwired: 2 in, 2 out]
              }
              frame "White Balance  **" {
                n187 = Index Array(array=w321, index=1) -> (element=w322:cluster{string[]})
                n188 = call <vilib>:"NT Read String.vi"("Name"=w324) -> ("String"=w323:string)  [unwired: 9 in, 1 out]
                n189 = Unbundle(w322) -> (w319:string[])
                n190 = Match First String(2:w319, 3:w323) -> (0:w318:i32)  [unwired: 1 out]
                n191 = property on="Test Ring" class="Ring (strict)"("Value"=w318, "Strings []"=w319) -> ()  [unwired: 2 in, 2 out]
                n192 = property on="Test Ring" class="Ring (strict)"("Visible"=TRUE) -> ()  [unwired: 2 in, 2 out]
                n193 = property on="Test Slider" class="Slide (strict)"("Visible"=FALSE) -> ()  [unwired: 2 in, 2 out]
              }
              frame "Exposure  **" {
                n194 = Index Array(array=w330, index=2) -> (element=w331:cluster{string[]})
                n195 = call <vilib>:"NT Read String.vi"("Name"=w333) -> ("String"=w332:string)  [unwired: 9 in, 1 out]
                n196 = Unbundle(w331) -> (w327:string[])
                n197 = Match First String(2:w327, 3:w332) -> (0:w328:i32)  [unwired: 1 out]
                n198 = property on="Test Ring" class="Ring (strict)"("Value"=w328, "Strings []"=w327) -> ()  [unwired: 2 in, 2 out]
                n199 = property on="Test Ring" class="Ring (strict)"("Visible"=TRUE) -> ()  [unwired: 2 in, 2 out]
                n200 = property on="Test Slider" class="Slide (strict)"("Visible"=FALSE) -> ()  [unwired: 2 in, 2 out]
              }
              frame "Exposure Priority  **" {
                n201 = Index Array(array=w339, index=3) -> (element=w340:cluster{string[]})
                n202 = call <vilib>:"NT Read String.vi"("Name"=w342) -> ("String"=w341:string)  [unwired: 9 in, 1 out]
                n203 = Unbundle(w340) -> (w336:string[])
                n204 = Match First String(2:w336, 3:w341) -> (0:w337:i32)  [unwired: 1 out]
                n205 = property on="Test Ring" class="Ring (strict)"("Value"=w337, "Strings []"=w336) -> ()  [unwired: 2 in, 2 out]
                n206 = property on="Test Ring" class="Ring (strict)"("Visible"=TRUE) -> ()  [unwired: 2 in, 2 out]
                n207 = property on="Test Slider" class="Slide (strict)"("Visible"=FALSE) -> ()  [unwired: 2 in, 2 out]
              }
              frame "Color Enable  **" {
                n208 = Index Array(array=w348, index=4) -> (element=w349:cluster{string[]})
                n209 = call <vilib>:"NT Read String.vi"("Name"=w351) -> ("String"=w350:string)  [unwired: 9 in, 1 out]
                n210 = Unbundle(w349) -> (w345:string[])
                n211 = Match First String(2:w345, 3:w350) -> (0:w346:i32)  [unwired: 1 out]
                n212 = property on="Test Ring" class="Ring (strict)"("Value"=w346, "Strings []"=w345) -> ()  [unwired: 2 in, 2 out]
                n213 = property on="Test Ring" class="Ring (strict)"("Visible"=TRUE) -> ()  [unwired: 2 in, 2 out]
                n214 = property on="Test Slider" class="Slide (strict)"("Visible"=FALSE) -> ()  [unwired: 2 in, 2 out]
              }
              frame Default {
                n215 = property on="Test Ring" class="Ring (strict)"("Visible"=FALSE) -> ()  [unwired: 2 in, 2 out]
                n216 = property on="Test Slider" class="Slide (strict)"("Visible"=FALSE) -> ()  [unwired: 2 in, 2 out]
              }
              frame "Brightness  **", "Color Level  **", "Compression  **", "FPS  **", "Sharpness  **" {
                n217 = call <vilib>:"NT Read Number.vi"("Name"=w357) -> ("Numeric"=w356:dbl)  [unwired: 9 in, 1 out]
                n218 = local write "Test Slider"(w356) -> ()
                n219 = property on="Test Slider" class="Slide (strict)"("Visible"=TRUE, "Scale.Maximum"=100.0 ("Scale.Range:Maximum")) -> ()  [unwired: 2 in, 2 out]
                n220 = property on="Test Ring" class="Ring (strict)"("Visible"=FALSE) -> ()  [unwired: 2 in, 2 out]
              }
            }
          }
        }
        n221 = property on="Progress" class="Clust (strict)"("Visible"=FALSE) -> ()  [unwired: 2 in, 2 out]
      }
      event "Test Name": Mouse Enter {
        # "Populate the ring with the list of tests"
        n222 = event-data() -> ()  [unwired: 1 in, 1 out]
        n223 = call <vilib>:"NT Read String Array.vi"("Name"="TestMode/TestList") -> ("String Array"=w365:string[])  [unwired: 9 in, 1 out]
        n224 = Build Array (concatenate)("Select the test to run...", w365) -> (w364:string[])
        n225 = property on="Test Name" class="Ring (strict)"("Strings []"=w364) -> ()  [unwired: 2 in, 2 out]
      }
      event "Test Name": Value Change {
        w367 = FALSE ("Visible")
        # "Tell the robot the test name to run"
        n226 = event-data() -> ("NewVal"=w371:u16)  [unwired: 1 in]
        n227 = property on="Test Name" class="Ring (strict)"() -> ("Strings []"=w372:string[])  [unwired: 2 in, 2 out]
        n228 = local write "Progress"(T6 {"Test Progress"=0, "Test Progress Text"=""} ("Progress")) -> ()
        n229 = Index Array(array=w372, index=w371) -> (element=w370:string)
        n230 = call <vilib>:"NT Write String.vi"("String"=w370, "Name"="TestMode/TestName") -> ()  [unwired: 9 in, 1 out]
        n231 = property on="Progress" class="Clust (strict)"("Visible"=TRUE) -> ()  [unwired: 2 in, 2 out]
        n232 = property on="Motor" class="Clust (strict)"("Visible"=w367) -> ()  [unwired: 2 in, 2 out]
        n233 = property on="Test Slider" class="Slide (strict)"("Visible"=w367) -> ()  [unwired: 2 in, 2 out]
        n234 = property on="On/Off" class="Bool (strict)"("Visible"=w367) -> ()  [unwired: 2 in, 2 out]
        n235 = property on="Rev/Fwd" class="Clust (strict)"("Visible"=w367) -> ()  [unwired: 2 in, 2 out]
        n236 = property on="Test Ring" class="Ring (strict)"("Visible"=w367) -> ()  [unwired: 2 in, 2 out]
      }
      event "Select Auto": Mouse Enter {
        # "Populate the combo box with the list of autonomous options"
        n237 = event-data() -> ()  [unwired: 1 in, 1 out]
        n238 = call <vilib>:"NT Read String Array.vi"("Name"="Auto List") -> ("String Array"=w374:string[])  [unwired: 9 in, 1 out]
        n239 = property on="Select Auto" class="CmbBox"("Strings[]"=w374) -> ()  [unwired: 2 in, 2 out]
      }
      event "Select Auto": Value Change {
        # "User modified the Auto Selection. Write to NT variable so robot knows."
        n240 = event-data() -> ("NewVal"=w377:string)  [unwired: 1 in]
        n241 = call <vilib>:"NT Write String.vi"("String"=w377, "Name"="Auto Selector") -> ()  [unwired: 9 in, 1 out]
      }
      event "Command Selection": Value Change {
        # "Get the params and show in table"
        n242 = event-data() -> ("NewVal"=w383:i32)  [unwired: 1 in]
        n243 = property on="Command Selection" class="MCListbox (strict)"() -> ("ItemNames"=w381:string[][])  [unwired: 2 in, 2 out]
        n244 = call <vilib>:"WPI_DashboardUpdate Command Params.vi"("NewVal"=w383, "Commands"=w381, "Param Tbl"=w382) -> ()  [unwired: 8 in, 1 out]
      }
      event "Execute Command": Value Change {
        # "Started one, Unique ID holds\nresponse"
        n245 = event-data() -> ()  [unwired: 1 in, 1 out]
        n246 = property on="Command Selection" class="MCListbox (strict)"() -> ("ItemNames"=w394:string[][])  [unwired: 2 in, 2 out]
        n247 = Index Array(array=w394, index (row)="Command Selection", index (col)=0) -> (element=w392:string)
        n248 = call <vilib>:"Invoke Commands.vi"("Command Params"="Command Params", "Function Name"=w392) -> ("Params"=w388:u8, "Started"=w387:bool)  [unwired: 7 in, 1 out]
        n249 = Array Subset(array="Command Params", length (row)=w388) -> (w389:string[][])  [unwired: 3 in]
        n250 = Select(t="Executing" ("Cmd Status"), s=w387, f="" ("Cmd Status")) -> (s? t:f=→"Cmd Status":string)
      }
      event "Command Selection": Double Click {
        n251 = event-data() -> ("Row"=w402:i32)  [unwired: 1 in]
        n252 = property on="Command Selection" class="MCListbox (strict)"() -> ("ItemNames"=w405:string[][])  [unwired: 2 in, 2 out]
        n253 = local read "Command Params"() -> (w401:string[][])
        n254 = Index Array(array=w405, index (row)=w402, index (col)=0) -> (element=w403:string)
        n255 = call <vilib>:"Invoke Commands.vi"("Command Params"=w401, "Function Name"=w403) -> ("Params"=w400:u8, "Started"=w395:bool)  [unwired: 7 in, 1 out]
        n256 = Array Subset(array=w401, length (row)=w400) -> (w399:string[][])  [unwired: 3 in]
        n257 = Select(t="Executing" ("Cmd Status"), s=w395, f="" ("Cmd Status")) -> (s? t:f=w396:string)
        n258 = local write "Cmd Status"(w396) -> ()
      }
      event "CheckList": Double Click {
        # "Shift clears all"
        # "Update symbols on the listbox"
        n259 = event-data() -> ("PlatMods.Shift"=w407:bool, "Row"=w409:i32)  [unwired: 1 in]
        n260 = case shown="True" w407 {
          tunnel: w409 -> [w413 _]
          tunnel: 1 -> [w412 _]
          frame False {
            n261 = property on="CheckList" class="LstBox (strict)"() -> ("Item Symbols"=w411:i32[])  [unwired: 2 in, 2 out]
            n262 = Replace Array Subset(array=w411, new element=w412, index=w413) -> (w410:i32[])
            n263 = property on="CheckList" class="LstBox (strict)"("Item Symbols"=w410) -> ()  [unwired: 2 in, 2 out]
          }
          frame True {
            w414 = 0 ("Top Row")
            n264 = property on="CheckList" class="LstBox (strict)"() -> ("Number of Rows"=w416:u32)  [unwired: 2 in, 2 out]
            n265 = Initialize Array(0, w416) -> (w415:i32[])
            n266 = property on="CheckList" class="LstBox (strict)"("Top Row"=w414, "Value"=w414, "Item Symbols"=w415) -> ()  [unwired: 2 in, 2 out]
          }
        }
      }
      event "CheckList": Key Down {
        # "Update symbols on the listbox\nLeft and right keys check and uncheck"
        n267 = event-data() -> ("VKey"=w420:T22)  [unwired: 1 in]
        n268 = case shown="\"Left\", \"Right\"" w420 {
          selector: w420 -> [w425 _]
          tunnel: eventvkey."Left" ("VKey") -> [w423 _]
          frame "Left", "Right" {
            n269 = Equal?(x=w423, y=w425) -> (x = y?=w424:bool)
            n270 = Select(t=0, s=w424, f=1) -> (s? t:f=w426:i32)
            n271 = property on="CheckList" class="LstBox (strict)"() -> ("Item Symbols"=w429:i32[])  [unwired: 2 in, 2 out]
            n272 = Replace Array Subset(array=w429, new element=w426, index="CheckList") -> (w428:i32[])
            n273 = property on="CheckList" class="LstBox (strict)"("Item Symbols"=w428) -> ()  [unwired: 2 in, 2 out]
          }
          frame Default {
          }
        }
      }
      event "Motor.Enable": Value Change {
        # "When the test mode otor enable helper is set, update that\ntree row item's value"
        n274 = event-data() -> ("NewVal"=w435:bool)  [unwired: 1 in]
        n275 = Unbundle("Motor") -> ("Value"=w434:dbl)  [unwired: 1 out]
        n276 = Select(t=w434, s=w435, f=0.0) -> (s? t:f=w432:dbl)
        n277 = call <vilib>:"NT Write Number.vi"("Numeric"=w432, "Name"=w431) -> ()  [unwired: 9 in, 1 out]
      }
      event "Test Slider": Value Change {
        # "When the test mode slider helper is set, update that\ntree row item's value"
        n278 = event-data() -> ("NewVal"=w438:dbl)  [unwired: 1 in]
        n279 = call <vilib>:"NT Write Number.vi"("Numeric"=w438, "Name"=w439) -> ()  [unwired: 9 in, 1 out]
      }
      event "On/Off": Value Change {
        # "When the test mode on/off helper value is set, update that\ntree row item's value"
        n280 = event-data() -> ("NewVal"=w443:bool)  [unwired: 1 in]
        n281 = Boolean To (0,1)(Boolean=w443) -> (0, 1=w442:i16)
        n282 = call <vilib>:"NT Write Number.vi"("Numeric"=w442, "Name"=w441) -> ()  [unwired: 9 in, 1 out]
      }
      event "Rev/Fwd": Value Change {
        # "When the test mode helper value for relays is set, update that\ntree row item's value"
        n283 = event-data() -> ("NewVal.Forward"=w451:bool, "NewVal.Reverse"=w450:bool)  [unwired: 1 in]
        n284 = Boolean To (0,1)(Boolean=w451) -> (0, 1=w447:i16)
        n285 = Boolean To (0,1)(Boolean=w450) -> (0, 1=w449:i16)
        n286 = Negate(x=w449) -> (-x=w448:i16)
        n287 = Add(x=w447, y=w448) -> (x+y=w446:i16)
        n288 = call <vilib>:"NT Write Number.vi"("Numeric"=w446, "Name"=w445) -> ()  [unwired: 9 in, 1 out]
      }
      event "Test Ring": Value Change {
        # "When a test mode helper value is selected from the ring,\nset the tree item's variable to the string value"
        n289 = event-data() -> ("NewVal"=w455:u16)  [unwired: 1 in]
        n290 = property on="Test Ring" class="Ring (strict)"() -> ("Strings []"=w456:string[])  [unwired: 2 in, 2 out]
        n291 = Index Array(array=w456, index=w455) -> (element=w454:string)
        n292 = call <vilib>:"NT Write String.vi"("String"=w454, "Name"=w453) -> ()  [unwired: 9 in, 1 out]
      }
      event "Rec Mode": Value Change {
        # "Update globals for recording mode and path to read log from.\nClear when logging and let NetworkTables set path for vision to\nuse."
        n293 = event-data() -> ("NewVal"=w467:enum32{"Stop", "Record", "Playback"})  [unwired: 1 in]
        n294 = global write "WPI_DashboardLogging Global.vi" "Logging Filename"(path "") -> ()
        n295 = global write "WPI_DashboardLogging Global.vi" "Recording"(w467) -> ()
        n296 = case shown="\"Playback\"" w467 {
          tunnel: w466 -> [_ w469 w478]
          tunnel: [_ _ w477] -> w464
          tunnel: [_ _ w476] -> _
          tunnel: w462 -> [_ _ w474]
          tunnel: cluster{i32, i32} {-250, 170} -> [_ _ w473]
          tunnel: [_ _ T23 {"Image Size"=TRUE, "Image Type"=TRUE, "Pixel Value"=TRUE, "ROI Information"=TRUE, "Zoom Factor"=FALSE} ("Image Information Shown:All Elements")] -> w457
          tunnel: [_ _ TRUE ("Zoom Factor")] -> w458
          tunnel: w460 -> [_ _ w470]
          frame Default {
          }
          frame "Stop", "Record" {
            # "Place Window too"
            n297 = invoke class="VI" method="FP.Close"(reference=w469) -> (reference out=w468:refnum<vi>)  [unwired: 2 in, 2 out]
            n298 = invoke class="VI" method="Abort VI"(reference=w468) -> ()  [unwired: 2 in, 3 out]
          }
          frame "Playback" {
            n299 = call "Open Playback Panel.vi"("Offset"=w473, "DB VI Ref"=w474, "Playback in"=w478) -> ("Playback out"=w475:refnum<vi>)  [unwired: 8 in]
            n300 = register-events(w475, w470) -> (reference out=w477:refnum<event-registration>, error out=w476:errorcluster)  [unwired: 2 in]
          }
        }
        n301 = property on="Camera Image Right" class="ImageControl"("Image Information Shown"=w457, "Image Information Visible"=w458) -> ()  [unwired: 2 in, 2 out]
        n302 = property on="Camera Image" class="ImageControl"("Image Information Shown"=w457, "Image Information Visible"=w458) -> ()  [unwired: 2 in, 2 out]
        n303 = call <vilib>:"WPI_DashboardNT Log FieldName Cache.vi"("Operation"=enum16{"Lookup/Add", "Index", "Clear"}."Clear") -> ()  [unwired: 8 in, 3 out]
      }
      event Panel Close {
        w480 = enum32{"Stop", "Record", "Playback"}."Stop" ("Rec Mode")
        # "Playback window has been closed, abort"
        n304 = event-data() -> ()  [unwired: 1 in, 4 out]
        n305 = local write "Rec Mode"(w480) -> ()
        n306 = global write "WPI_DashboardLogging Global.vi" "Recording"(w480) -> ()
      }
      event Panel Close {
        # "Abort playback window and ourself"
        n307 = event-data() -> ()  [unwired: 1 in, 4 out]
        n308 = invoke class="VI" method="FP.Close"(reference=w484) -> (reference out=w483:refnum<vi>)  [unwired: 2 in, 2 out]
        n309 = invoke class="VI" method="Abort VI"(reference=w483) -> (error out=w482:errorcluster)  [unwired: 2 in, 2 out]
        n310 = invoke class="VI" method="Abort VI"(error in=w482) -> ()  [unwired: 2 in, 3 out]
      }
      event User Event {
        n311 = event-data() -> ("IDs"=w491:cluster{"RPC field ID":u16, "Unique ID":u16}, "String"=w490:string)  [unwired: 1 in]
        n312 = Bundle("IDs"=w491, "String"=w490) -> (w489:T9)  [unwired: 1 in]
        n313 = call <vilib>:"Retrieve RPC Response.vi"("RPC Response"=w489) -> ("Output"=w487:string[][])  [unwired: 10 in]
        n314 = Build Array (concatenate)(w485, w487) -> (w486:string[][])
        n315 = local write "Command Params"(w486) -> ()
        n316 = local write "Cmd Status"("" ("Cmd Status")) -> ()
      }
      event "Tree": Double Click {
        n317 = event-data() -> ("PlatMods"=w497:T26, "Tag"=w494:string)  [unwired: 1 in]
        n318 = Unbundle(w497) -> ("Shift"=w496:bool)  [unwired: 4 out]
        n319 = String Subset(string=w494, length (rest)=1 ("length (rest)")) -> (substring=w493:string)  [unwired: 1 in]
        n320 = Not(x=w496) -> (.not. x?=w495:bool)
        n321 = case shown="\"/\"" w493 {
          tunnel: w494 -> [_ w500]
          tunnel: w495 -> [_ w499]
          frame Default {
          }
          frame "/" {
            n322 = call <vilib>:"NT Update Persistence.vi"("Persistence"=w499, "Name"=w500) -> ()  [unwired: 9 in, 1 out]
          }
        }
      }
    }
  }
  n323 = while {
    tunnel: w69 -> [w502]
    i -> [w505]
    stop <- FALSE stop-if-true
    n324 = Wait (ms)(milliseconds to wait=u32 100) -> ()  [unwired: 1 out]
    n325 = case shown="\"Playback\"" "Rec Mode" {
      tunnel: w505 -> [_ _ w520]
      tunnel: [u32 2829099 ("Base Color") u32 11141120 ("Target Color") w509] -> w501
      frame "Stop", Default {
        # "Reset the color, extra updates don't cost much"
      }
      frame "Record" {
      }
      frame "Playback" {
        # "Playback"
        n326 = Quotient & Remainder(x=w520, y=u32 50 ("milliseconds to wait")) -> (x-y*floor(x/y)=w516:u32)  [unwired: 1 out]
        n327 = Divide(x=w516, y=u32 50 ("milliseconds to wait")) -> (x/y=w513:dbl)
        n328 = Multiply(x=6.283185307179586, y=w513) -> (x*y=w518:dbl)
        n329 = Sine(x=w518) -> (sin(x)=w517:dbl)
        n330 = Absolute Value(x=w517) -> (abs(x)=w510:dbl)
        n331 = call "Interpolate RGB Color.vi"("Proportion"=w510, "Target Color"=u32 30976, "Base Color"=u32 2829099) -> ("Result Color"=w509:u32)  [unwired: 8 in]
      }
    }
    n332 = property class="Pane"(reference=w502, "PaneColor"=w501) -> ()  [unwired: 1 in, 2 out]
  }
  n333 = local write "Dashboard Tab"(T2."Drive" ("Dashboard Tab")) -> ()
  n334 = property on="On/Off" class="Bool (strict)"("Visible"=w40) -> ()  [unwired: 2 in, 2 out]
  n335 = property on="Motor" class="Clust (strict)"("Visible"=w40) -> ()  [unwired: 2 in, 2 out]
  n336 = property on="Progress" class="Clust (strict)"("Visible"=w40) -> ()  [unwired: 2 in, 2 out]
  n337 = property on="Test Ring" class="Ring (strict)"("Visible"=w40) -> ()  [unwired: 2 in, 2 out]
  n338 = property on="Rev/Fwd" class="Clust (strict)"("Visible"=w40) -> ()  [unwired: 2 in, 2 out]
  n339 = while {
    tunnel: u16 1741 ("timeout ms (25000)") -> [w522]
    stop <- FALSE stop-if-true
    n340 = TCP Create Listener(10:w522) -> (0:w521:errorcluster, 3:w523:refnum<k5>)  [unwired: 4 in, 1 out]
    n341 = case shown="No Error" w521 {
      selector: w521 -> [w525 _]
      tunnel: w523 -> [w526 _]
      frame No Error {
        n342 = while {
          tunnel: w526 -> [w529]
          tunnel: w525 -> [w528]
          stop <- FALSE stop-if-true
          n343 = TCP Wait On Listener(8:w528, 11:w529) -> (0:w530:errorcluster, 4:w531:refnum<k5>)  [unwired: 2 in, 3 out]
          n344 = local write "TCP"(w531) -> ()
          n345 = case shown="No Error" w530 {
            frame No Error {
            }
            frame Error {
              n346 = Wait (ms)(milliseconds to wait=u32 1000) -> ()  [unwired: 1 out]
            }
          }
        }
      }
      frame Error {
        n347 = Wait (ms)(milliseconds to wait=u32 1000) -> ()  [unwired: 1 out]
      }
    }
  }
  n348 = local write "Command Selection"(u16 0 ("milliseconds to wait")) -> ()
  n349 = local write "Command Params"(string[][] [] ("Command Params")) -> ()
  n350 = global write "WPI_DashboardLogging Global.vi" "Recording"(w63) -> ()
  n351 = local write "Rec Mode"(w63) -> ()
  n352 = call <vilib>:"NT Write String.vi"("String"="Select Auto", "Name"="Auto Selector") -> ()  [unwired: 9 in, 1 out]
